vi "Nelder-Mead_alignment.vi"() -> ()   [LabVIEW 2024]
uses:
  5b59031f-b1ff-41af-80a7-e72a33ebffa1.vi
  <vilib>/Array/Sort 2D Array - Pop Stack.vi
  <vilib>/Array/Sort 2D Array - Push Stack.vi
  5b59031f-b1ff-41af-80a7-e72a33ebffa1.vi/269d4b3b-47f5-49e3-8884-44851e4dd9d5.vi
  5b59031f-b1ff-41af-80a7-e72a33ebffa1.vi/6d99389c-673d-4efb-bf33-19b32bcf4cf8.vi
panel:
  out "# pts tested":i32
  out "Full-Output_pts_tested":dbl[][][](array[numeric])
  out "i":i32
  out "x_c":dbl[](array[numeric])
  out "x_e":dbl[](array[numeric])
  out "x_o":dbl[](array[numeric])
  out "x_r":dbl[](array[numeric])
  in  "sigma":dbl=0.5 format="%#_13g"
  in  "rho":dbl=0.5 format="%#_13g"
  in  "gamma":dbl=2.0 format="%#_13g"
  in  "alpha":dbl=1.0 format="%#_13g"
  out "Optimized Loc":dbl[](array[numeric])
  in  "stop":bool
  out "test_locs":dbl[][](array[numeric])
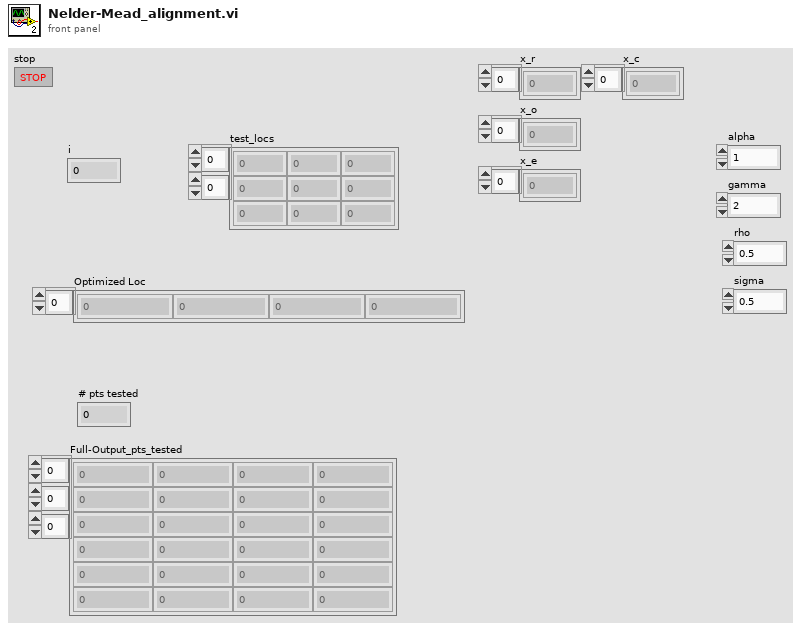
[diagram p1: front panel]
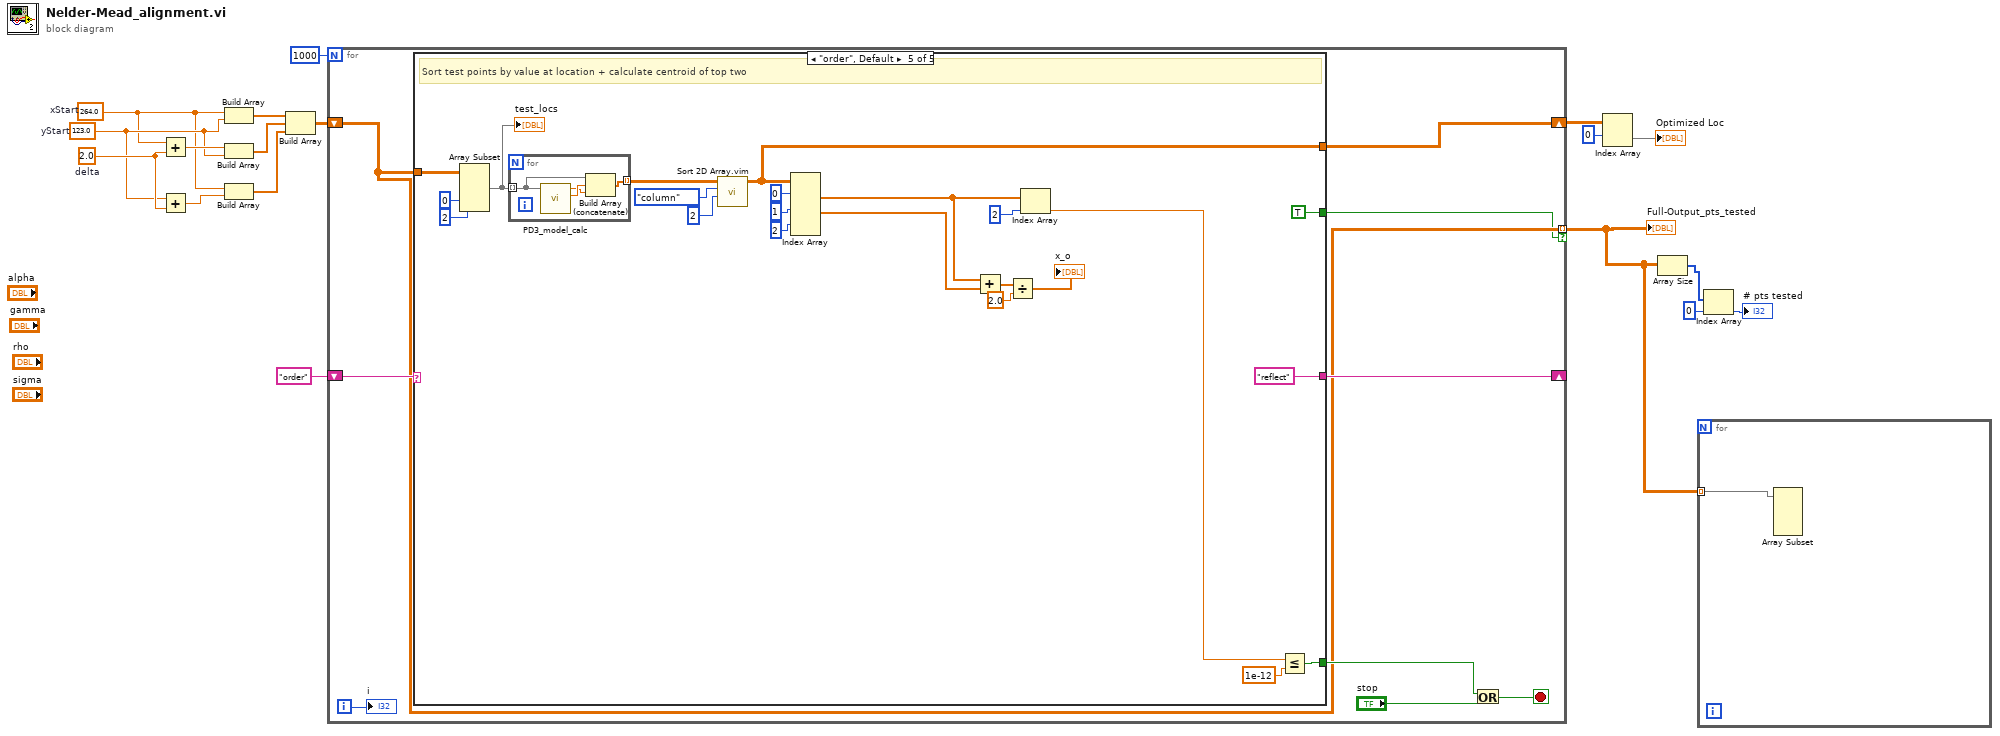
[diagram p0: block diagram]
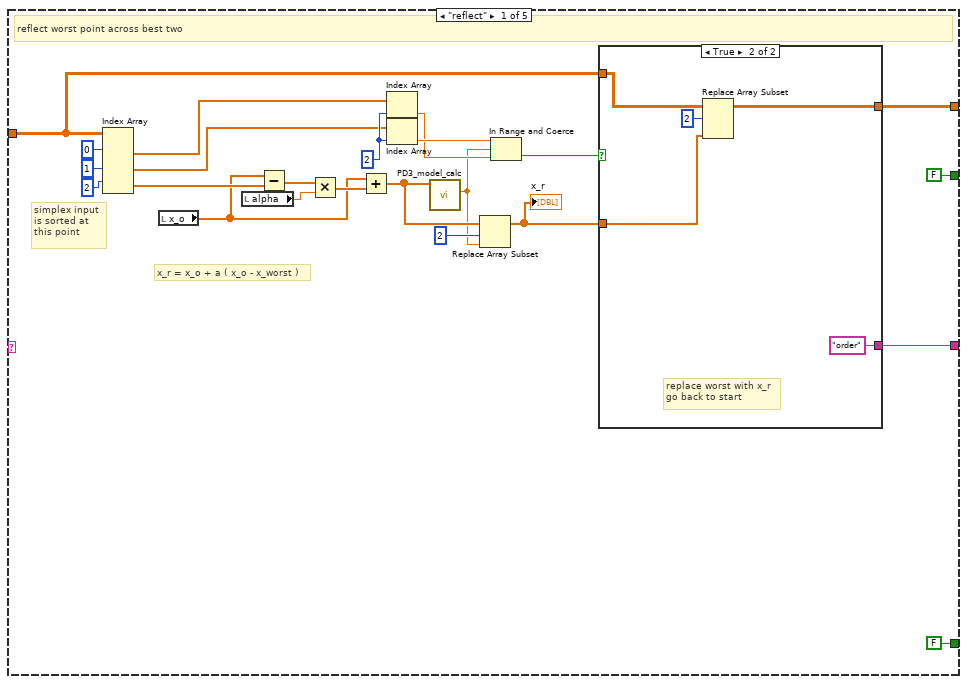
[diagram p2: hidden frame]
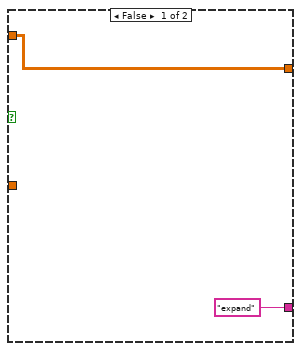
[diagram p3: hidden frame]
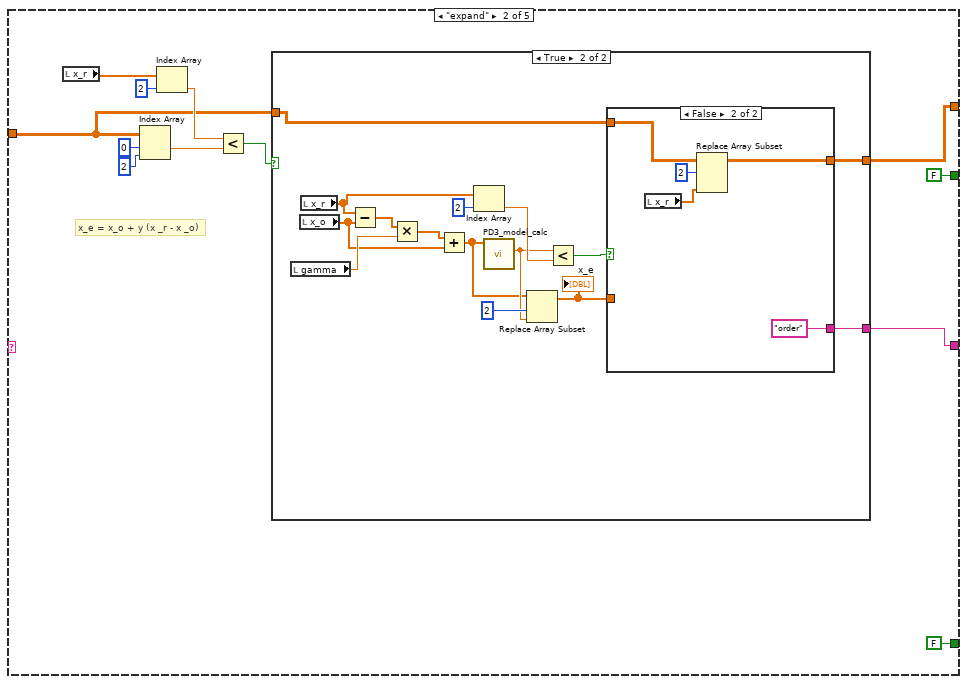
[diagram p4: hidden frame]
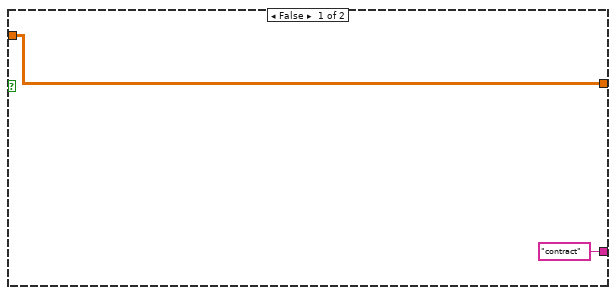
[diagram p5: hidden frame]
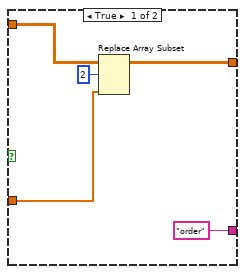
[diagram p6: hidden frame]
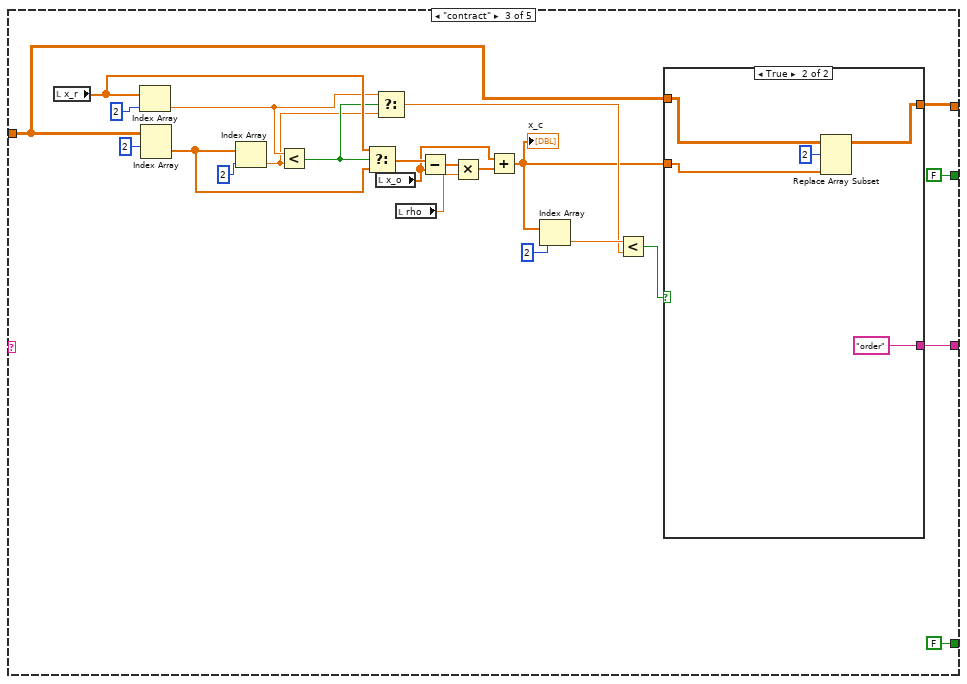
[diagram p7: hidden frame]
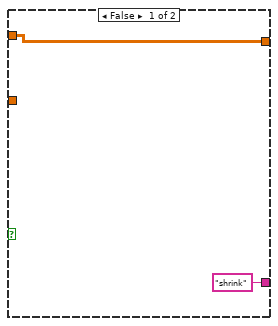
[diagram p8: hidden frame]
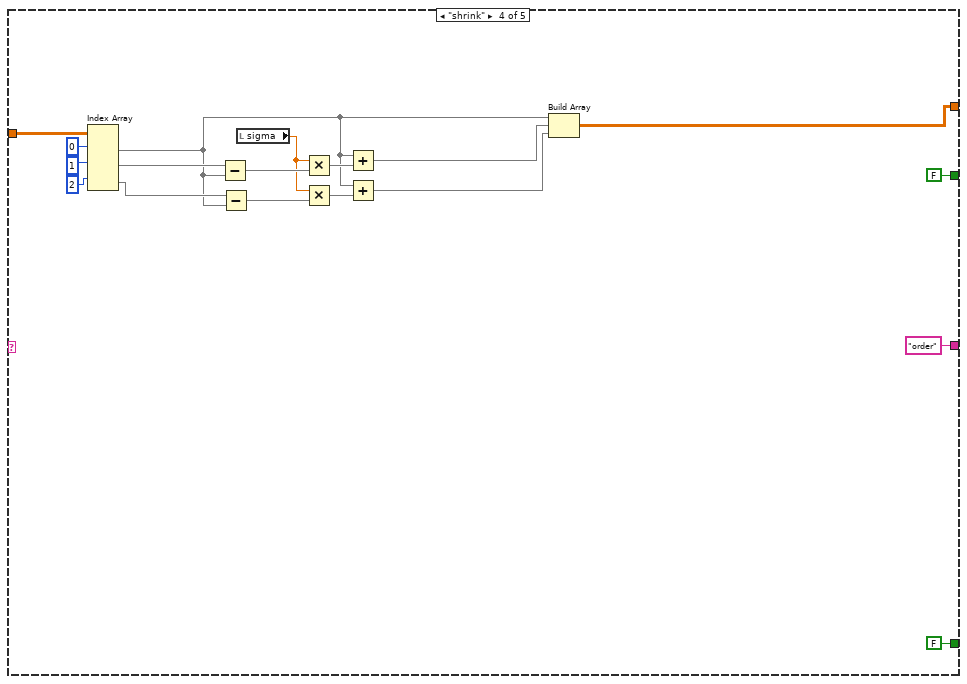
[diagram p9: hidden frame]
diagram:
  w12 = 123.0  # yStart
  w11 = 264.0  # xStart
  w13 = 2.0  # delta
  n1 = Add(x=w11, y=w13) -> (x+y=w14:dbl)
  n2 = Add(x=w12, y=w13) -> (x+y=w15:dbl)
  n3 = Build Array(w11, w12) -> (w16:dbl[])
  n4 = Build Array(w14, w12) -> (w17:dbl[])
  n5 = Build Array(w11, w15) -> (w18:dbl[])
  n6 = Build Array(w16, w17, w18) -> (w10:dbl[][])
  n7 = for {
    N: 1000 -> [_]
    shift-right: [w21] -> w9
    shift-left: w10 -> [w20]
    shift-right: [w22] -> _
    shift-left: "order" -> [w25]
    tunnel: [w20] -> w6 mode=indexing if=w19
    i -> [w23]
    stop <- w27 stop-if-true
    n8 = case shown="\"order\", Default" w25 {
      tunnel: w20 -> [w32 w62 w99 w142 w154]
      tunnel: [FALSE FALSE FALSE FALSE w158] -> w26
      tunnel: [w31 w61 w100 w128 w152] -> w21
      tunnel: [w33 w60 w101 "order" "reflect"] -> w22
      tunnel: [FALSE FALSE FALSE FALSE TRUE] -> w19
      frame "reflect" {
        w43 = 2 ("index")
        # "simplex input\nis sorted at\nthis point"
        # "x_r = x_o + a ( x_o - x_worst )"
        # "reflect worst point across best two"
        n9 = Index Array(array=w32, index (row) #1=0 ("index (row)"), index (row) #2=1 ("index (row)"), index (row) #3=2 ("index (row)")) -> (element #1=w42:dbl[], element #2=w41:dbl[], element #3=w44:dbl[])  [unwired: 3 in]
        n10 = local read "x_o"() -> (w34:dbl[])
        n11 = local read "alpha"() -> (w48:dbl)
        n12 = Subtract(x=w34, y=w44) -> (x-y=w49:dbl[])
        n13 = Multiply(x=w49, y=w48) -> (x*y=w47:dbl[])
        n14 = Add(x=w34, y=w47) -> (x+y=w37:dbl[])
        n15 = Index Array(array=w42, index=w43) -> (element=w39:dbl)
        n16 = Index Array(array=w41, index=w43) -> (element=w40:dbl)
        n17 = call "PD3_model_calc.vi"("pos_in"=w37) -> ("Param_Out"=w35:dbl)  [unwired: 9 in, 1 out]
        n18 = Replace Array Subset(array=w37, new element=w35, index=2) -> (w29:dbl[])
        "x_r" <- w29
        n19 = In Range and Coerce(upper limit=w40, x=w35, lower limit=w39) -> (In Range?=w38:bool)  [unwired: 1 out]
        n20 = case shown="True" w38 {
          tunnel: ["expand" "order"] -> w33
          tunnel: w32 -> [w51 w57]
          tunnel: [w51 w54] -> w31
          tunnel: w29 -> [_ w55]
          frame False {
          }
          frame True {
            # "replace worst with x_r\ngo back to start"
            n21 = Replace Array Subset(array=w57, new element=w55, index (row)=2) -> (w54:dbl[][])  [unwired: 1 in]
          }
        }
      }
      frame "expand" {
        # "x_e = x_o + y (x _r - x _o)"
        n22 = local read "x_r"() -> (w67:dbl[])
        n23 = Index Array(array=w62, index (row)=0, index (col)=2 ("disabled index (col)")) -> (element=w65:dbl)
        n24 = Index Array(array=w67, index=2) -> (element=w64:dbl)
        n25 = Less?(x=w64, y=w65) -> (x < y?=w63:bool)
        n26 = case shown="True" w63 {
          tunnel: w62 -> [w71 w78]
          tunnel: [w71 w73] -> w61
          tunnel: ["contract" w72] -> w60
          frame False {
          }
          frame True {
            n27 = local read "gamma"() -> (w85:dbl)
            n28 = local read "x_o"() -> (w83:dbl[])
            n29 = local read "x_r"() -> (w82:dbl[])
            n30 = Subtract(x=w82, y=w83) -> (x-y=w86:dbl[])
            n31 = Multiply(x=w86, y=w85) -> (x*y=w84:dbl[])
            n32 = Add(x=w84, y=w83) -> (x+y=w75:dbl[])
            n33 = Index Array(array=w82, index=2) -> (element=w80:dbl)
            n34 = call "PD3_model_calc.vi"("pos_in"=w75) -> ("Param_Out"=w76:dbl)  [unwired: 9 in, 1 out]
            n35 = Replace Array Subset(array=w75, new element=w76, index=2) -> (w74:dbl[])
            "x_e" <- w74
            n36 = Less?(x=w76, y=w80) -> (x < y?=w79:bool)
            n37 = case shown="False" w79 {
              tunnel: w78 -> [w90 w95]
              tunnel: w74 -> [w89 _]
              tunnel: [w88 w94] -> w73
              tunnel: ["order" "order"] -> w72
              frame True {
                n38 = Replace Array Subset(array=w90, new element=w89, index (row)=2) -> (w88:dbl[][])  [unwired: 1 in]
              }
              frame False {
                n39 = local read "x_r"() -> (w92:dbl[])
                n40 = Replace Array Subset(array=w95, new element=w92, index (row)=2) -> (w94:dbl[][])  [unwired: 1 in]
              }
            }
          }
        }
      }
      frame "contract" {
        n41 = local read "x_r"() -> (w115:dbl[])
        n42 = Index Array(array=w115, index=2) -> (element=w107:dbl)
        n43 = Index Array(array=w99, index (row)=2) -> (element=w114:dbl[])  [unwired: 1 in]
        n44 = Index Array(array=w114, index=2) -> (element=w106:dbl)
        n45 = Less?(x=w107, y=w106) -> (x < y?=w108:bool)
        n46 = Select(t=w115, s=w108, f=w114) -> (s? t:f=w113:dbl[])
        n47 = Select(t=w107, s=w108, f=w106) -> (s? t:f=w103:dbl)
        n48 = local read "x_o"() -> (w109:dbl[])
        n49 = local read "rho"() -> (w111:dbl)
        n50 = Subtract(x=w113, y=w109) -> (x-y=w112:dbl[])
        n51 = Multiply(x=w112, y=w111) -> (x*y=w110:dbl[])
        n52 = Add(x=w109, y=w110) -> (x+y=w98:dbl[])
        "x_c" <- w98
        n53 = Index Array(array=w98, index=2) -> (element=w104:dbl)
        n54 = Less?(x=w104, y=w103) -> (x < y?=w102:bool)
        n55 = case shown="True" w102 {
          tunnel: ["shrink" "order"] -> w101
          tunnel: [w120 w122] -> w100
          tunnel: w99 -> [w120 w124]
          tunnel: w98 -> [_ w123]
          frame False {
          }
          frame True {
            n56 = Replace Array Subset(array=w124, new element=w123, index (row)=2) -> (w122:dbl[][])  [unwired: 1 in]
          }
        }
      }
      frame "shrink" {
        n57 = Index Array(array=w142, index (row) #1=0 ("index (row)"), index (row) #2=1 ("index (row)"), index (row) #3=2 ("index (row)")) -> (element #1=w131:dbl[], element #2=w138:dbl[], element #3=w137:dbl[])  [unwired: 3 in]
        n58 = Subtract(x=w138, y=w131) -> (x-y=w135:dbl[])
        n59 = Subtract(x=w137, y=w131) -> (x-y=w136:dbl[])
        n60 = local read "sigma"() -> (w134:dbl)
        n61 = Multiply(x=w134, y=w135) -> (x*y=w133:dbl[])
        n62 = Multiply(x=w134, y=w136) -> (x*y=w132:dbl[])
        n63 = Add(x=w131, y=w133) -> (x+y=w130:dbl[])
        n64 = Add(x=w131, y=w132) -> (x+y=w129:dbl[])
        n65 = Build Array(w131, w130, w129) -> (w128:dbl[][])
      }
      frame "order", Default {
        # "Sort test points by value at location + calculate centroid of top two"
        n66 = Array Subset(array=w154, index (col)=0 ("index"), length (col)=2 ("length")) -> (w155:dbl[][])  [unwired: 2 in]
        "test_locs" <- w155
        n67 = for {
          tunnel: w155 -> [w168] mode=indexing
          tunnel: [w169] -> w166 mode=indexing
          n68 = call "PD3_model_calc.vi"("pos_in"=w168) -> ("Param_Out"=w170:dbl, "I_out"=w167:dbl)  [unwired: 9 in]
          n69 = Build Array (concatenate)(w168, w170, w167) -> (w169:dbl[])
        }
        n70 = call "Sort 2D Array.vim"("index"=2, "dimension to index (column)"=enum16{"column", "row"}."column", "2D array"=w166) -> ("sorted 2D array"=w152:dbl[][])  [unwired: 7 in, 1 out]
        n71 = Index Array(array=w152, index (row) #1=0 ("index (row)"), index (row) #2=1 ("index (row)"), index (row) #3=2 ("index (row)")) -> (element #1=w151:dbl[], element #2=w150:dbl[])  [unwired: 3 in, 1 out]
        n72 = Add(x=w151, y=w150) -> (x+y=w148:dbl[])
        n73 = Divide(x=w148, y=2.0) -> (x/y=→"x_o":dbl[])
        n74 = Index Array(array=w151, index=2) -> (element=w153:dbl)
        n75 = Less Or Equal?(x=w153, y=1e-12) -> (x <= y?=w158:bool)
      }
    }
    n76 = Or(x=w26, y="stop") -> (x .or. y?=w27:bool)
    "i" <- w23
  }
  "Full-Output_pts_tested" <- w6
  n77 = Index Array(array=w9, index (row)=0) -> (element=→"Optimized Loc":dbl[])  [unwired: 1 in]
  n78 = Array Size(array=w6) -> (size(s)=w3:i32[])
  n79 = for {
    tunnel: w6 -> [w171] mode=indexing
    n80 = Array Subset(array=w171) -> ()  [unwired: 4 in, 1 out]
  }
  n81 = Index Array(array=w3, index=0) -> (element=→"# pts tested":i32)
